vi "Data File Processing UI Add Type Message.vi"(0 "queue in":refnum<queue>, 5 "Msg":T1, 11 "error in":errorcluster) -> (4 "queue out":refnum<queue>, 15 "error out":errorcluster)   [LabVIEW 2012]
uses:
  Data File Processing UI Message Define.ctl
  Data File Processing UI Message Type Define.ctl
panel:
  in  "time out":i32=-1
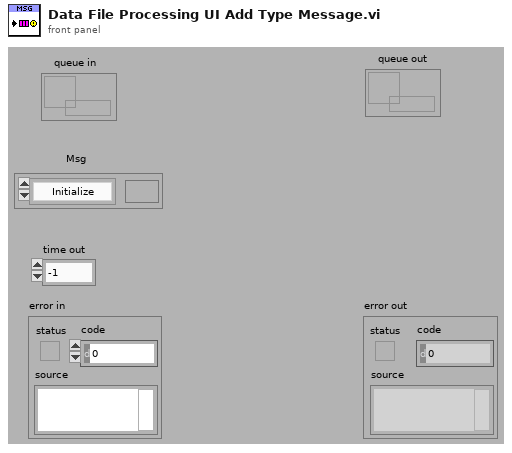
[diagram p1: front panel]
types:
  T1 = typedef "Data File Processing UI Message Define.ctl" = cluster{"data":variant, "type":T2}
  T2 = typedef "Data File Processing UI Message Type Define.ctl" = enum32{"Initialize", "SleepThread", "ErrorHandler", "NoEvent", "PreExit", "Exit", "----Action----", "OpenFile", "ReadAllCompute", "SaveFile", "RedrawGraph", "SelectChannel"}
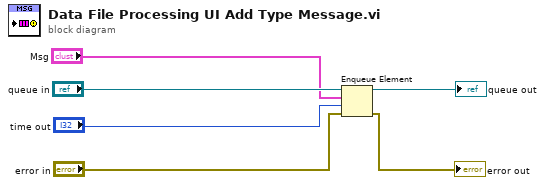
[diagram p0: block diagram]
diagram:
  n1 = Enqueue Element(queue="queue in", element="Msg", timeout in ms (-1)="time out", error in (no error)="error in") -> (queue out=→"queue out":refnum<queue>, error out=→"error out":errorcluster)  [unwired: 1 out]
